vi "Actual Replot.vi"(8 "error in (no error)":errorcluster, 11 "Plot in":refnum<class "Plot.lvclass">) -> (0 "error out":errorcluster, 3 "Plot out":refnum<class "Plot.lvclass">)   [LabVIEW 2016, in "Plot.lvclass"]
uses:
  Plot.lvclass
  Plot.lvclass/Plot.ctl
  Write Replot request.vi
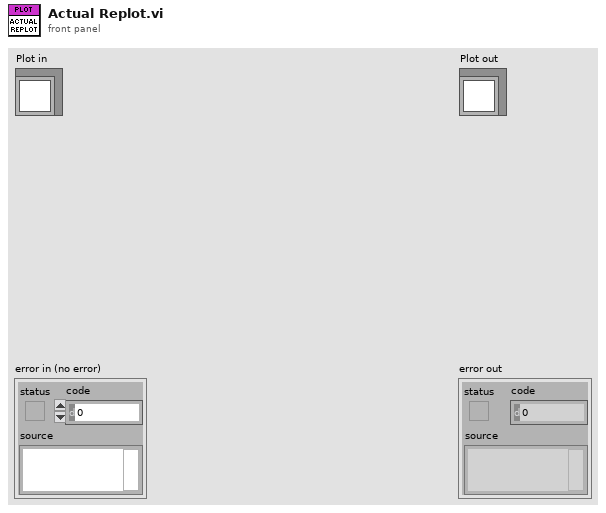
[diagram p1: front panel]
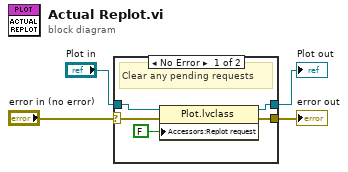
[diagram p0: block diagram]
diagram:
  n1 = case shown="No Error" "error in (no error)" {
    selector: "error in (no error)" -> [w9 w11]
    tunnel: [w8 w11] -> w3
    tunnel: [w6 w10] -> w1
    tunnel: "Plot in" -> [w7 w10]
    frame No Error {
      # "Clear any pending requests"
      n2 = property class="Plot.lvclass"(reference=w7, error in=w9, "Accessors:Replot request"=FALSE) -> (reference out=w6:refnum<class "Plot.lvclass">, error out=w8:errorcluster)
    }
    frame Error {
    }
  }
  "error out" <- w3
  "Plot out" <- w1
